vi "Unflatten.vi"(8 "error in (no error)":errorcluster, 11 "Magnetic Field in":refnum<class "Magnetic Field.lvclass">) -> (0 "error out":errorcluster, 3 "Magnetic Field out":refnum<class "Magnetic Field.lvclass">)   [LabVIEW 2009, in "Magnetic Field.lvclass"]
uses:
  Magnetic Field.lvclass
  Scanner/Scanner.lvclass
  Global/File Locations.vi
  Magnetic Field.lvclass/Magnetic Field.ctl
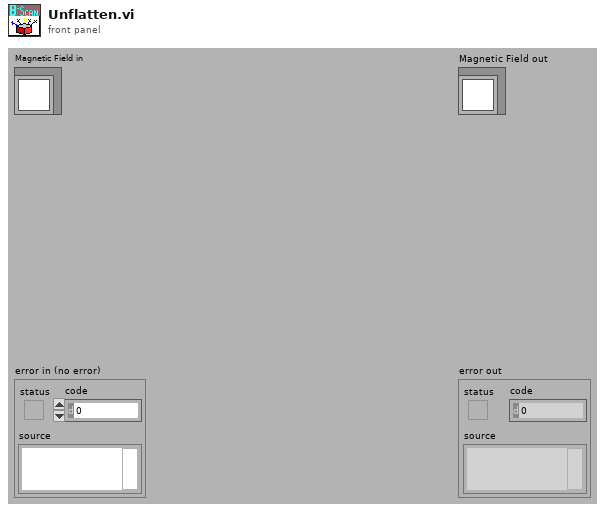
[diagram p1: front panel]
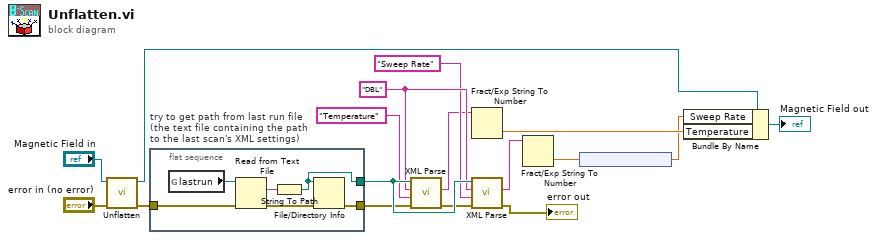
[diagram p0: block diagram]
diagram:
  w12 = "DBL"
  n1 = call-parent "Unflatten.vi"("error in (no error)"="error in (no error)", "Scanner in"="Magnetic Field in") -> ("error out"=w4:errorcluster, "Scanner out"=w17:refnum<class "Magnetic Field.lvclass">)  [unwired: 8 in]
  n2 = flat-sequence "try to get path from last run file\n(the text file containing the path\nto the last scan's XML settings)" {
    tunnel: [w23] -> w13
    tunnel: [w19] -> w9
    tunnel: w4 -> [w18]
    frame #0 {
      n3 = global read "File Locations.vi" "lastrun"() -> (w21:path)
      n4 = Read from Text File(file (use dialog)=w21, error in=w18) -> (text=w22:string, error out=w20:errorcluster)  [unwired: 4 out]
      n5 = String To Path(string=w22) -> (path=w23:path)
      n6 = File/Directory Info(path=w23, error in=w20) -> (error out=w19:errorcluster)  [unwired: 6 out]
    }
  }
  n7 = call "XML Parse.vi"("error in (no error)"=w9, "Name String"="Temperature", "Type String"=w12, "Path"=w13) -> ("error out"=w8:errorcluster, "String Out"=w7:string)  [unwired: 6 in]
  n8 = Fract/Exp String To Number(string=w7) -> (number=w3:dbl)  [unwired: 3 in, 1 out]
  n9 = call "XML Parse.vi"("error in (no error)"=w8, "Name String"="Sweep Rate", "Type String"=w12, "Path"=w13) -> ("error out"=→"error out":errorcluster, "String Out"=w6:string)  [unwired: 6 in]
  n10 = Fract/Exp String To Number(string=w6) -> (number=w5:dbl)  [unwired: 3 in, 1 out]
  n11 = node(w5) -> (w2:dbl[unit])
  n12 = Bundle By Name(cluster=w17, "Sweep Rate"=w2, "Temperature"=w3) -> (→"Magnetic Field out":refnum<class "Magnetic Field.lvclass">)
